vi "Get Cursor Position.vi"() -> (3 "cursor position":cluster{"x":i16, "y":i16})   [LabVIEW 2020, in "MacroAssert.lvlib" / "Winsys.lvlib"]
doc: "This VI returns the mouse position in screen coordinates."
uses:
  Winsys.lvlib
  user32.dll
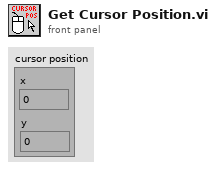
[diagram p1: front panel]
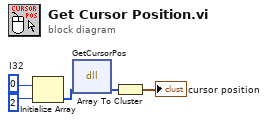
[diagram p0: block diagram]
diagram:
  w5 = 0  # I32
  n1 = Initialize Array(w5, 2) -> (w3:i32[])
  n2 = dll-call lib="user32.dll" fn="GetCursorPos"("POINT"=w3) -> ("POINT"=w2:i32[])  [unwired: 3 in, 3 out]
  n3 = Array To Cluster(array=w2) -> (cluster=→"cursor position":cluster{"POINT[0]":i32, "POINT[1]":i32})
